vi "RTS Individual Station Timers.vi"(4 "Relay Number":u8, 6 "Station #":u8, 8 "error in (no error)":errorcluster, 10 "Open Door Timer (s)":dbl, 11 "Reset Timer?":bool) -> (0 "error out":errorcluster, 2 "Times Up?":bool, 3 "Elapsed Time (sec)":dbl)   [LabVIEW 2016]
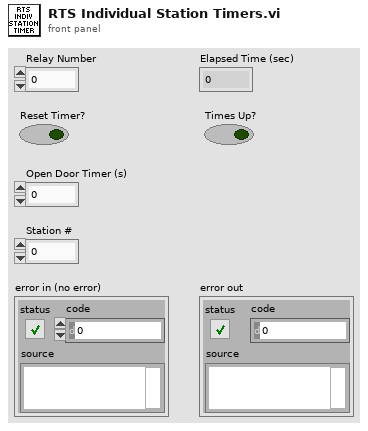
[diagram p1: front panel]
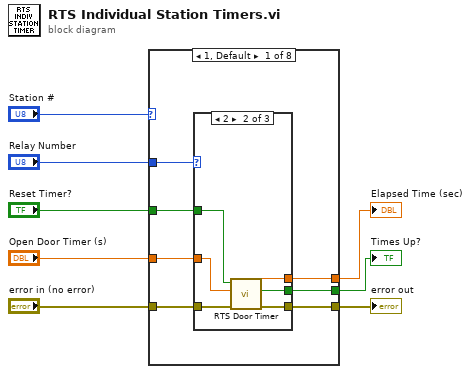
[diagram p0: block diagram]
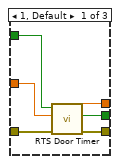
[diagram p2: hidden frame]
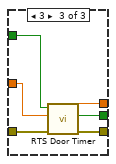
[diagram p3: hidden frame]
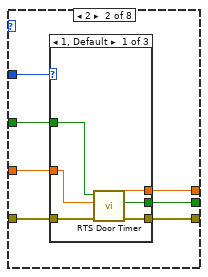
[diagram p4: hidden frame]
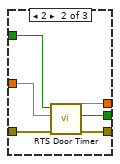
[diagram p5: hidden frame]
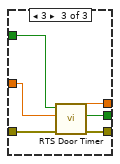
[diagram p6: hidden frame]
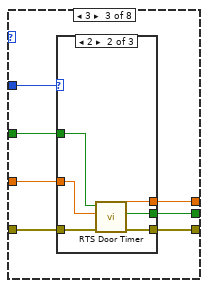
[diagram p7: hidden frame]
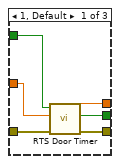
[diagram p8: hidden frame]
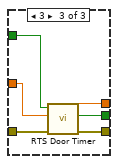
[diagram p9: hidden frame]
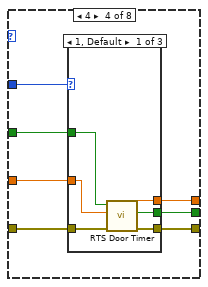
[diagram p10: hidden frame]
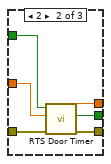
[diagram p11: hidden frame]
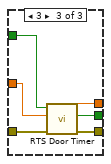
[diagram p12: hidden frame]
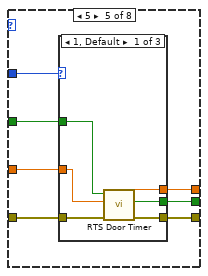
[diagram p13: hidden frame]
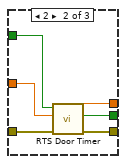
[diagram p14: hidden frame]
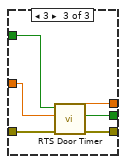
[diagram p15: hidden frame]
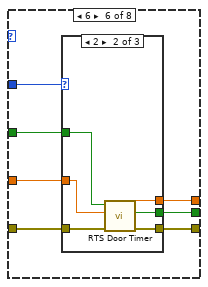
[diagram p16: hidden frame]
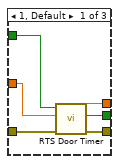
[diagram p17: hidden frame]
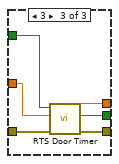
[diagram p18: hidden frame]
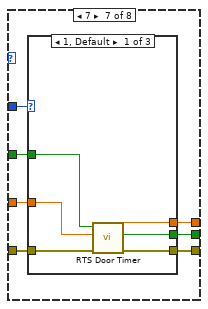
[diagram p19: hidden frame]
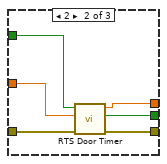
[diagram p20: hidden frame]
diagram:
  n1 = case shown="1, Default" "Station #" {
    tunnel: [w15 w35 w61 w87 w111 w138 w161 w186] -> w1
    tunnel: [w14 w34 w60 w86 w110 w137 w160 w185] -> w2
    tunnel: [w13 w39 w64 w88 w112 w139 w164 w189] -> w3
    tunnel: "error in (no error)" -> [w12 w40 w65 w89 w113 w140 w165 w190]
    tunnel: "Reset Timer?" -> [w11 w36 w63 w85 w115 w136 w163 w188]
    tunnel: "Open Door Timer (s)" -> [w10 w37 w62 w84 w114 w135 w162 w187]
    tunnel: "Relay Number" -> [w9 w38 w59 w90 w109 w134 w159 w184]
    frame 1, Default {
      n2 = case shown="2" w9 {
        tunnel: [w21 w22 w29] -> w15
        tunnel: [w20 w23 w28] -> w14
        tunnel: [w19 w26 w32] -> w13
        tunnel: w12 -> [w18 w27 w33]
        tunnel: w11 -> [w17 w25 w31]
        tunnel: w10 -> [w16 w24 w30]
        frame 1, Default {
          n3 = call "RTS Door Timer.vi"("Error In"=w18, "Time Limit (sec)"=w16, "Reset Timer?"=w17) -> ("Error Out"=w19:errorcluster, "Times Up?"=w20:bool, "Elapsed Time (sec)"=w21:dbl)  [unwired: 6 in]
        }
        frame 2 {
          n4 = call "RTS Door Timer.vi"("Error In"=w27, "Time Limit (sec)"=w24, "Reset Timer?"=w25) -> ("Error Out"=w26:errorcluster, "Times Up?"=w23:bool, "Elapsed Time (sec)"=w22:dbl)  [unwired: 6 in]
        }
        frame 3 {
          n5 = call "RTS Door Timer.vi"("Error In"=w33, "Time Limit (sec)"=w30, "Reset Timer?"=w31) -> ("Error Out"=w32:errorcluster, "Times Up?"=w28:bool, "Elapsed Time (sec)"=w29:dbl)  [unwired: 6 in]
        }
      }
    }
    frame 2 {
      n6 = case shown="1, Default" w38 {
        tunnel: [w46 w47 w54] -> w35
        tunnel: [w45 w48 w53] -> w34
        tunnel: [w44 w51 w57] -> w39
        tunnel: w40 -> [w43 w52 w58]
        tunnel: w36 -> [w42 w50 w56]
        tunnel: w37 -> [w41 w49 w55]
        frame 1, Default {
          n7 = call "RTS Door Timer.vi"("Error In"=w43, "Time Limit (sec)"=w41, "Reset Timer?"=w42) -> ("Error Out"=w44:errorcluster, "Times Up?"=w45:bool, "Elapsed Time (sec)"=w46:dbl)  [unwired: 6 in]
        }
        frame 2 {
          n8 = call "RTS Door Timer.vi"("Error In"=w52, "Time Limit (sec)"=w49, "Reset Timer?"=w50) -> ("Error Out"=w51:errorcluster, "Times Up?"=w48:bool, "Elapsed Time (sec)"=w47:dbl)  [unwired: 6 in]
        }
        frame 3 {
          n9 = call "RTS Door Timer.vi"("Error In"=w58, "Time Limit (sec)"=w55, "Reset Timer?"=w56) -> ("Error Out"=w57:errorcluster, "Times Up?"=w53:bool, "Elapsed Time (sec)"=w54:dbl)  [unwired: 6 in]
        }
      }
    }
    frame 3 {
      n10 = case shown="2" w59 {
        tunnel: [w71 w72 w79] -> w61
        tunnel: [w70 w73 w78] -> w60
        tunnel: [w69 w76 w82] -> w64
        tunnel: w65 -> [w68 w77 w83]
        tunnel: w63 -> [w67 w75 w81]
        tunnel: w62 -> [w66 w74 w80]
        frame 1, Default {
          n11 = call "RTS Door Timer.vi"("Error In"=w68, "Time Limit (sec)"=w66, "Reset Timer?"=w67) -> ("Error Out"=w69:errorcluster, "Times Up?"=w70:bool, "Elapsed Time (sec)"=w71:dbl)  [unwired: 6 in]
        }
        frame 2 {
          n12 = call "RTS Door Timer.vi"("Error In"=w77, "Time Limit (sec)"=w74, "Reset Timer?"=w75) -> ("Error Out"=w76:errorcluster, "Times Up?"=w73:bool, "Elapsed Time (sec)"=w72:dbl)  [unwired: 6 in]
        }
        frame 3 {
          n13 = call "RTS Door Timer.vi"("Error In"=w83, "Time Limit (sec)"=w80, "Reset Timer?"=w81) -> ("Error Out"=w82:errorcluster, "Times Up?"=w78:bool, "Elapsed Time (sec)"=w79:dbl)  [unwired: 6 in]
        }
      }
    }
    frame 4 {
      n14 = case shown="1, Default" w90 {
        tunnel: [w96 w97 w104] -> w87
        tunnel: [w95 w98 w103] -> w86
        tunnel: [w94 w101 w107] -> w88
        tunnel: w89 -> [w93 w102 w108]
        tunnel: w85 -> [w92 w100 w106]
        tunnel: w84 -> [w91 w99 w105]
        frame 1, Default {
          n15 = call "RTS Door Timer.vi"("Error In"=w93, "Time Limit (sec)"=w91, "Reset Timer?"=w92) -> ("Error Out"=w94:errorcluster, "Times Up?"=w95:bool, "Elapsed Time (sec)"=w96:dbl)  [unwired: 6 in]
        }
        frame 2 {
          n16 = call "RTS Door Timer.vi"("Error In"=w102, "Time Limit (sec)"=w99, "Reset Timer?"=w100) -> ("Error Out"=w101:errorcluster, "Times Up?"=w98:bool, "Elapsed Time (sec)"=w97:dbl)  [unwired: 6 in]
        }
        frame 3 {
          n17 = call "RTS Door Timer.vi"("Error In"=w108, "Time Limit (sec)"=w105, "Reset Timer?"=w106) -> ("Error Out"=w107:errorcluster, "Times Up?"=w103:bool, "Elapsed Time (sec)"=w104:dbl)  [unwired: 6 in]
        }
      }
    }
    frame 5 {
      n18 = case shown="1, Default" w109 {
        tunnel: [w121 w122 w129] -> w111
        tunnel: [w120 w123 w128] -> w110
        tunnel: [w119 w126 w132] -> w112
        tunnel: w113 -> [w118 w127 w133]
        tunnel: w115 -> [w117 w125 w131]
        tunnel: w114 -> [w116 w124 w130]
        frame 1, Default {
          n19 = call "RTS Door Timer.vi"("Error In"=w118, "Time Limit (sec)"=w116, "Reset Timer?"=w117) -> ("Error Out"=w119:errorcluster, "Times Up?"=w120:bool, "Elapsed Time (sec)"=w121:dbl)  [unwired: 6 in]
        }
        frame 2 {
          n20 = call "RTS Door Timer.vi"("Error In"=w127, "Time Limit (sec)"=w124, "Reset Timer?"=w125) -> ("Error Out"=w126:errorcluster, "Times Up?"=w123:bool, "Elapsed Time (sec)"=w122:dbl)  [unwired: 6 in]
        }
        frame 3 {
          n21 = call "RTS Door Timer.vi"("Error In"=w133, "Time Limit (sec)"=w130, "Reset Timer?"=w131) -> ("Error Out"=w132:errorcluster, "Times Up?"=w128:bool, "Elapsed Time (sec)"=w129:dbl)  [unwired: 6 in]
        }
      }
    }
    frame 6 {
      n22 = case shown="2" w134 {
        tunnel: [w146 w147 w154] -> w138
        tunnel: [w145 w148 w153] -> w137
        tunnel: [w144 w151 w157] -> w139
        tunnel: w140 -> [w143 w152 w158]
        tunnel: w136 -> [w142 w150 w156]
        tunnel: w135 -> [w141 w149 w155]
        frame 1, Default {
          n23 = call "RTS Door Timer.vi"("Error In"=w143, "Time Limit (sec)"=w141, "Reset Timer?"=w142) -> ("Error Out"=w144:errorcluster, "Times Up?"=w145:bool, "Elapsed Time (sec)"=w146:dbl)  [unwired: 6 in]
        }
        frame 2 {
          n24 = call "RTS Door Timer.vi"("Error In"=w152, "Time Limit (sec)"=w149, "Reset Timer?"=w150) -> ("Error Out"=w151:errorcluster, "Times Up?"=w148:bool, "Elapsed Time (sec)"=w147:dbl)  [unwired: 6 in]
        }
        frame 3 {
          n25 = call "RTS Door Timer.vi"("Error In"=w158, "Time Limit (sec)"=w155, "Reset Timer?"=w156) -> ("Error Out"=w157:errorcluster, "Times Up?"=w153:bool, "Elapsed Time (sec)"=w154:dbl)  [unwired: 6 in]
        }
      }
    }
    frame 7 {
      n26 = case shown="1, Default" w159 {
        tunnel: [w171 w172 w179] -> w161
        tunnel: [w170 w173 w178] -> w160
        tunnel: [w169 w176 w182] -> w164
        tunnel: w165 -> [w168 w177 w183]
        tunnel: w163 -> [w167 w175 w181]
        tunnel: w162 -> [w166 w174 w180]
        frame 1, Default {
          n27 = call "RTS Door Timer.vi"("Error In"=w168, "Time Limit (sec)"=w166, "Reset Timer?"=w167) -> ("Error Out"=w169:errorcluster, "Times Up?"=w170:bool, "Elapsed Time (sec)"=w171:dbl)  [unwired: 6 in]
        }
        frame 2 {
          n28 = call "RTS Door Timer.vi"("Error In"=w177, "Time Limit (sec)"=w174, "Reset Timer?"=w175) -> ("Error Out"=w176:errorcluster, "Times Up?"=w173:bool, "Elapsed Time (sec)"=w172:dbl)  [unwired: 6 in]
        }
        frame 3 {
          n29 = call "RTS Door Timer.vi"("Error In"=w183, "Time Limit (sec)"=w180, "Reset Timer?"=w181) -> ("Error Out"=w182:errorcluster, "Times Up?"=w178:bool, "Elapsed Time (sec)"=w179:dbl)  [unwired: 6 in]
        }
      }
    }
    frame 8 {
      n30 = case shown="1, Default" w184 {
        tunnel: [w196 w197 w204] -> w186
        tunnel: [w195 w198 w203] -> w185
        tunnel: [w194 w201 w207] -> w189
        tunnel: w190 -> [w193 w202 w208]
        tunnel: w188 -> [w192 w200 w206]
        tunnel: w187 -> [w191 w199 w205]
        frame 1, Default {
          n31 = call "RTS Door Timer.vi"("Error In"=w193, "Time Limit (sec)"=w191, "Reset Timer?"=w192) -> ("Error Out"=w194:errorcluster, "Times Up?"=w195:bool, "Elapsed Time (sec)"=w196:dbl)  [unwired: 6 in]
        }
        frame 2 {
          n32 = call "RTS Door Timer.vi"("Error In"=w202, "Time Limit (sec)"=w199, "Reset Timer?"=w200) -> ("Error Out"=w201:errorcluster, "Times Up?"=w198:bool, "Elapsed Time (sec)"=w197:dbl)  [unwired: 6 in]
        }
        frame 3 {
          n33 = call "RTS Door Timer.vi"("Error In"=w208, "Time Limit (sec)"=w205, "Reset Timer?"=w206) -> ("Error Out"=w207:errorcluster, "Times Up?"=w203:bool, "Elapsed Time (sec)"=w204:dbl)  [unwired: 6 in]
        }
      }
    }
  }
  "error out" <- w3
  "Times Up?" <- w2
  "Elapsed Time (sec)" <- w1
